vi "Wait For Lock.vi"(10 "timeout (100 ms)":i32=100, 11 "UniqueName in":refnum<class "UniqueName.lvclass">) -> (2 "Locked":bool, 3 "UniqueName out":refnum<class "UniqueName.lvclass">)   [LabVIEW 2014, in "UniqueName.lvlib" / "UniqueName.lvclass"]
uses:
  UniqueName.lvclass
  Command.ctl
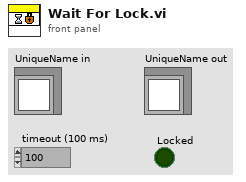
[diagram p1: front panel]
types:
  T1 = typedef "UniqueName.lvlib/UniqueName.lvclass/Command.ctl" = enum16{"Get", "Get All", "Set", "Delete", "Get Status", "Init", "Reserve Ownership", "Release Ownership", "Lock", "Unlock"}
  T2 = typedef "UniqueName.lvlib/UniqueName.lvclass/RegistryStatus.ctl" = cluster{"Registry Configuration":T3, "Registry Owned":bool, "Write-Protected":bool, "Owned":bool, "Released":bool, "Locked":bool, "Unlocked":bool}
  T3 = typedef "UniqueName.lvlib/UniqueName.lvclass/RegistryConfiguration.ctl" = cluster{"Delimiter":refnum<class "Delimiter.lvclass">, "RandomStringGenerator":refnum<class "RandomStringGenerator.lvclass">, "UniquenessCriteria":refnum<class "UniquenessCriteria.lvclass">, "StringIncrement":refnum<class "StringIncrementAlgorithm.lvclass">}
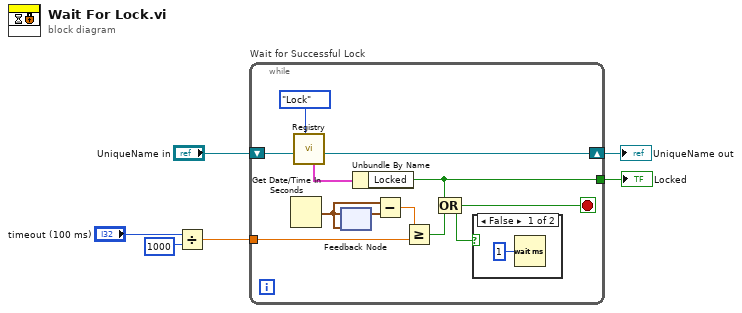
[diagram p0: block diagram]
diagram:
  n1 = Divide(x="timeout (100 ms)", y=1000) -> (x/y=w4:dbl)
  n2 = while "Wait for Successful Lock" {
    tunnel: [w13] -> w1
    tunnel: w4 -> [w15]
    shift-right: [w8] -> w5
    shift-left: "UniqueName in" -> [w9]
    stop <- w7 stop-if-true
    n3 = Get Date/Time In Seconds() -> (seconds since 1Jan1904=w12:timestamp)
    n4 = call "Registry.vi"("Command (Get)"=Command."Lock", "UniqueName Object (Set)"=w9) -> ("Returned Object"=w8:refnum<class "UniqueName.lvclass">, "Registry Status"=w16:T2)  [unwired: 5 in, 3 out]
    n5 = feedback-in #1(w12) -> ()
    n6 = feedback #1(w12) -> (w11:timestamp)
    n7 = Unbundle By Name(w16) -> ("Locked"=w13:bool)
    n8 = Subtract(x=w12, y=w11) -> (x-y=w10:dbl)
    n9 = Greater Or Equal?(x=w10, y=w15) -> (x >= y?=w14:bool)
    n10 = Compound Arithmetic op=OR(w13, w14) -> (w7:bool)
    n11 = case shown="False" w7 {
      frame False {
        n12 = Wait (ms)(milliseconds to wait=u32 1) -> ()  [unwired: 1 out]
      }
      frame True {
      }
    }
  }
  "UniqueName out" <- w5
  "Locked" <- w1
